vi "CC FITS Get FITS Name.vi"(11 "Full Name":string) -> (2 "ok?":bool, 3 "FITS Hdr Name":string)   [LabVIEW 2024]
panel:
  in  "Cancel Button":bool
  in  "OK Button":bool
  in  "FITS Name":string
  # "FITS name must be <= 8 letters with no spaces or special characters"
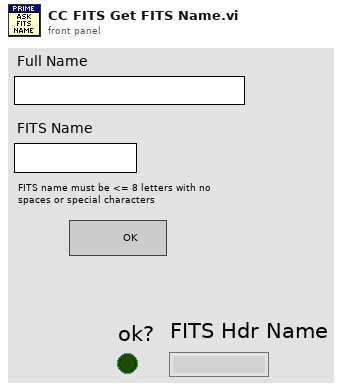
[diagram p1: front panel]
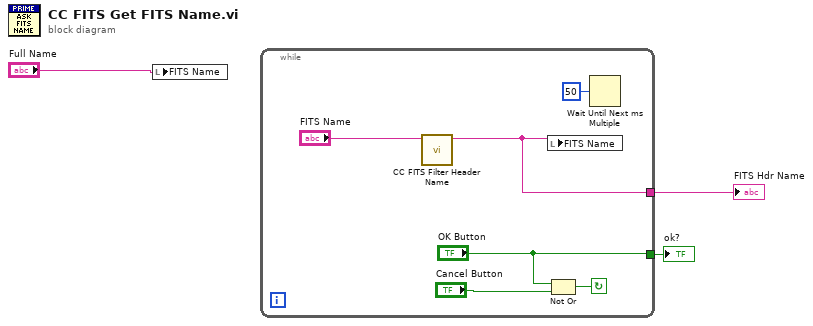
[diagram p0: block diagram]
diagram:
  n1 = local write "FITS Name"("Full Name") -> ()
  n2 = while {
    tunnel: ["OK Button"] -> w1
    tunnel: [w4] -> w2
    stop <- w8 continue-if-true
    n3 = call "CC FITS Filter Header Name.vi"("FITS Name In"="FITS Name") -> ("FITS Name Out"=w4:string)  [unwired: 9 in, 1 out]
    n4 = local write "FITS Name"(w4) -> ()
    n5 = Not Or(1:"Cancel Button", 2:"OK Button") -> (0:w8:bool)
    n6 = Wait Until Next ms Multiple(millisecond multiple=u32 50) -> ()  [unwired: 1 out]
  }
  "FITS Hdr Name" <- w2
  "ok?" <- w1
